vi "Instr Panel.vi"() -> ()   [LabVIEW 2009]
uses:
  Instruments/DAQ/DAQmx Analog.lvclass
  Instruments/Function Generator/Function Generator.lvclass
  Global/Flags.vi
  Main.vi
  Instruments/Utility Classes/Instrument/Instrument.lvclass
  File IO/File IO.lvclass
  Instruments/LCD/LCD Retarder.lvclass
  Instruments/Lockin/Lockin SR830.lvclass
  Instruments/Spectrometer/Spectrometer Triax 550.lvclass
  Instruments/Microwave/Microwave.lvclass
  Instruments/Pulse Gen/Pulse Generator.lvclass
  Instruments/Photon Counter/Photon Counter SR400.lvclass
  Instruments/Magnet/Power Supply/Power Supply.lvclass
panel:
  in  "Frequent\nReading":bool
  out "Find instruments (auto)":bool
  out "Status array":T1(array[cluster])
  in  "controlFMsweep":bool
  in  "Photon Counter":bool
  out "readtime":u32 caption="Read Time"
  in  "LDcontrol":bool
  in  "FGcontrol":bool
  in  "MWcontrol":bool
  in  "searchGPIB":bool
  in  "GPIB Comm.":bool
  in  "Find Instruments":bool
  in  "etchLD":bool
  in  "Open Driver":bool
  out "instrchecking":bool caption="Reading"
  in  "chop":bool
  in  "center-span":bool
  out "active":bool caption="Active"
  out "done":bool
  in  "exit":bool
  in  "Pulse Gen":bool
  in  "Magnet":bool
  in  "gotoLCD":bool
  in  "gotospect":bool
  # "On"
  # "Off"
  # "ms"
  # "Instruments Array"
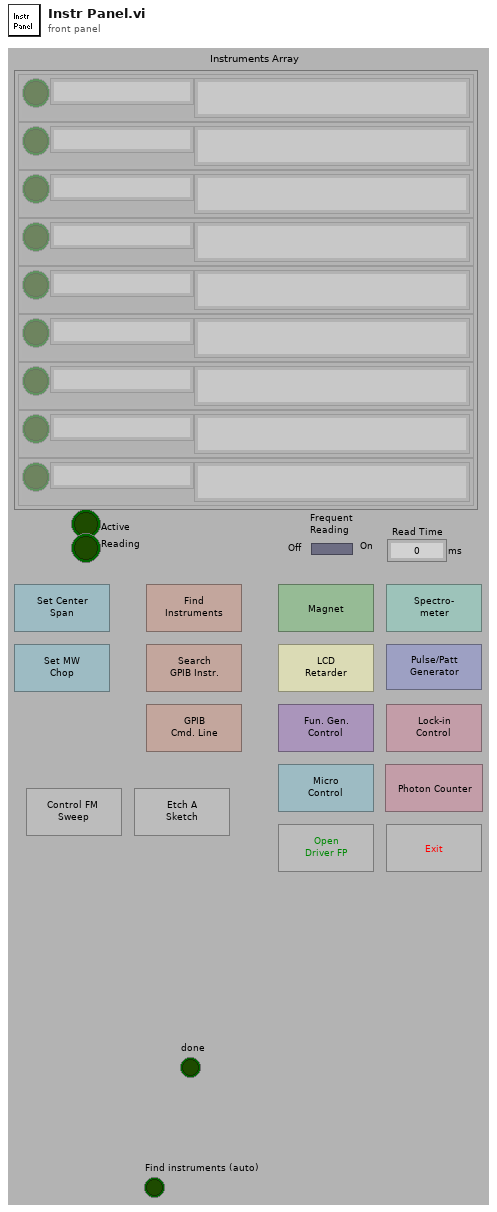
[diagram p1: front panel]
types:
  T1 = cluster{"On?":bool, "Name":string, "Status":string}[]
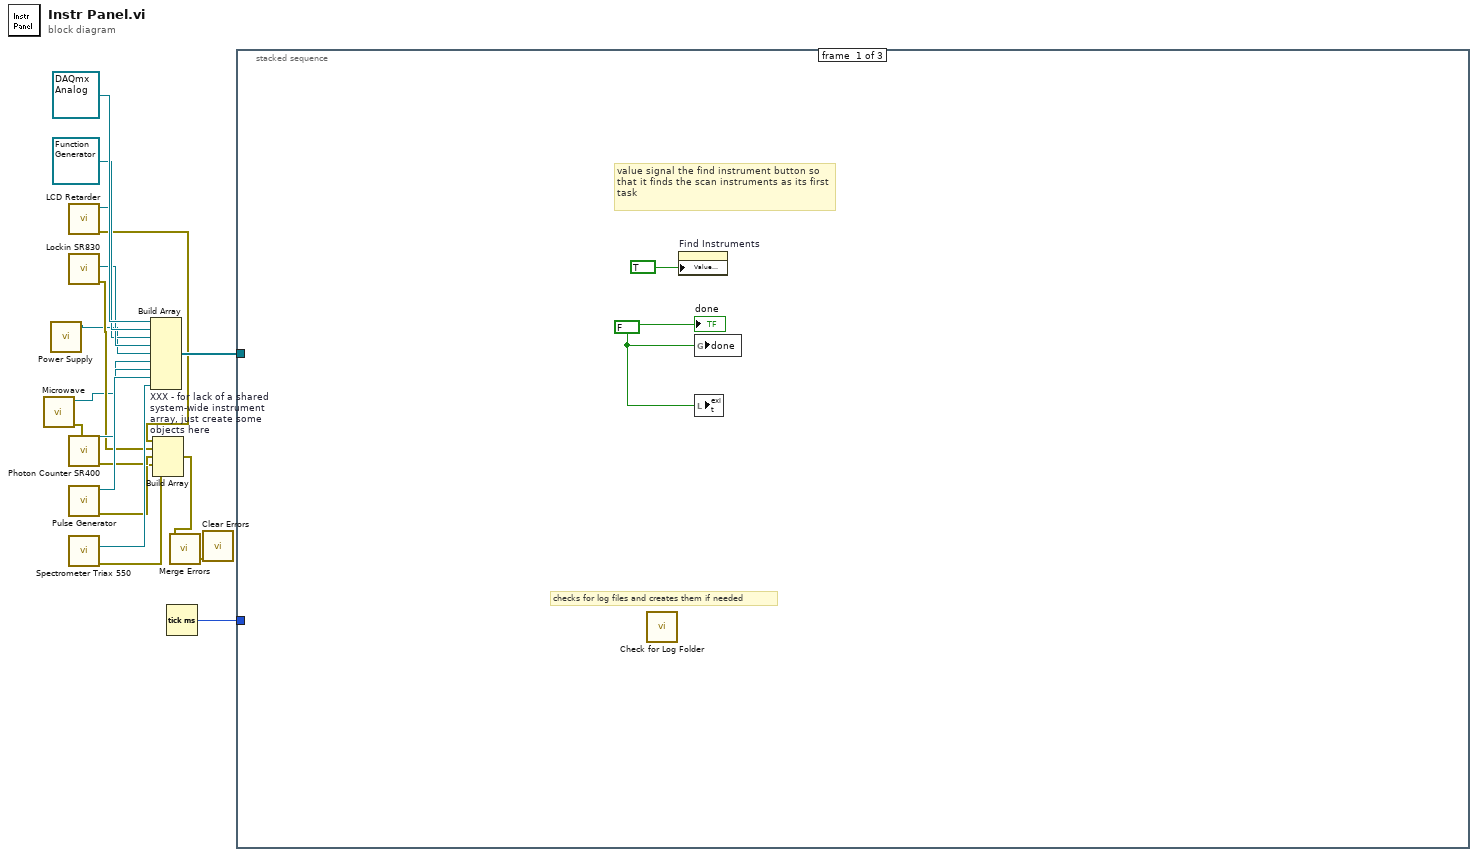
[diagram p0: block diagram]
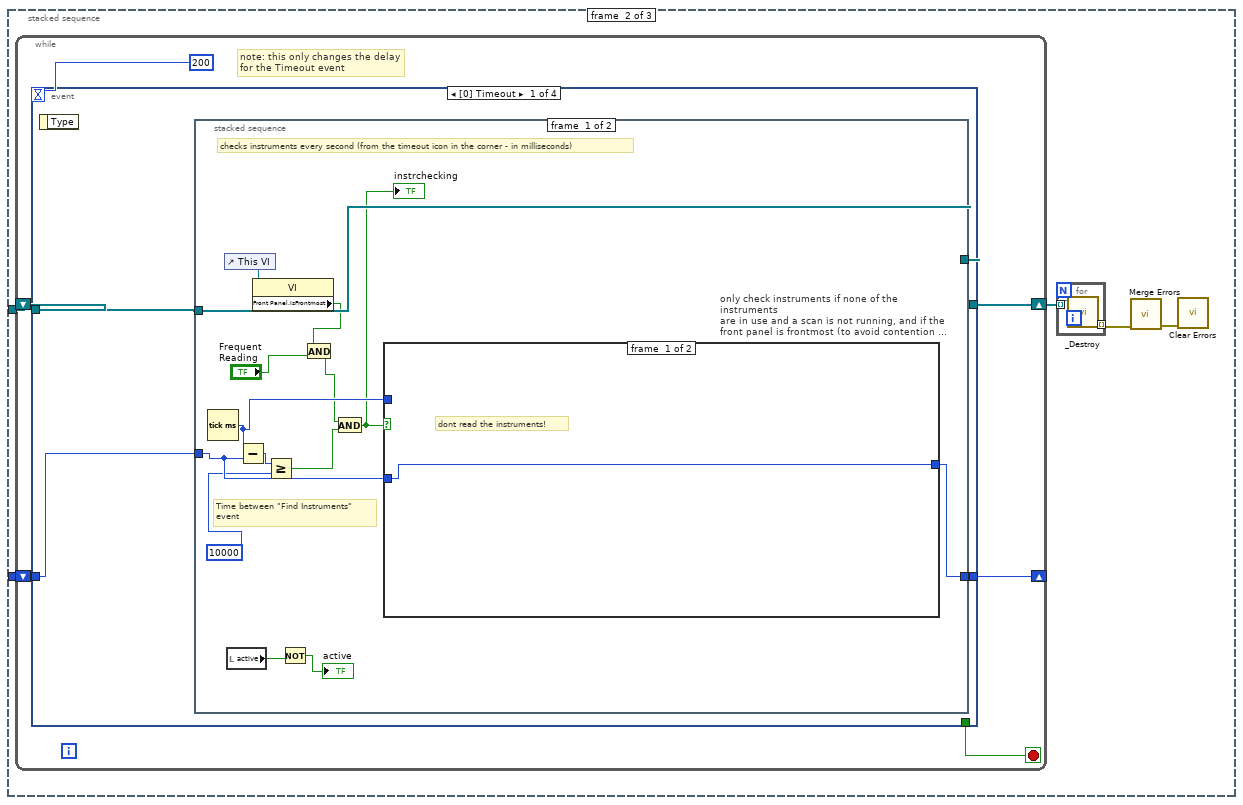
[diagram p2: hidden frame]
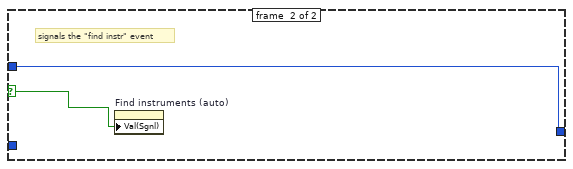
[diagram p3: hidden frame]
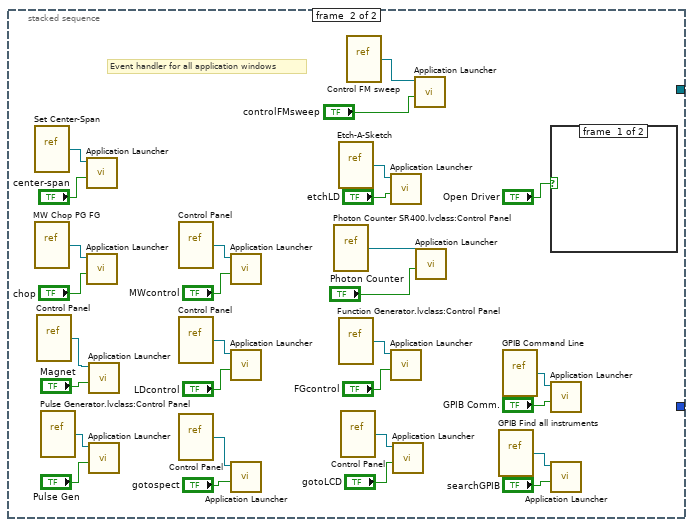
[diagram p4: hidden frame]
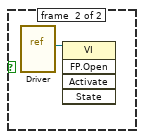
[diagram p5: hidden frame]
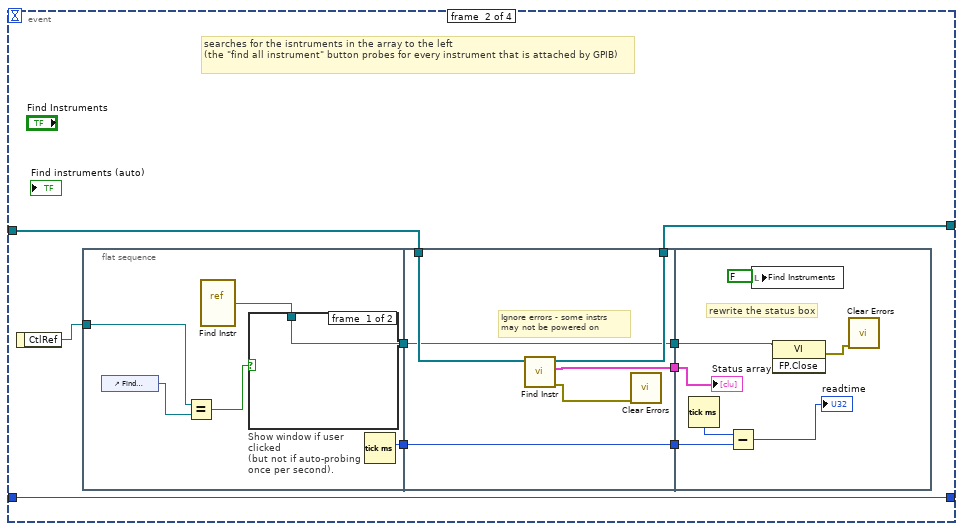
[diagram p6: hidden frame]
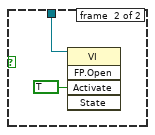
[diagram p7: hidden frame]
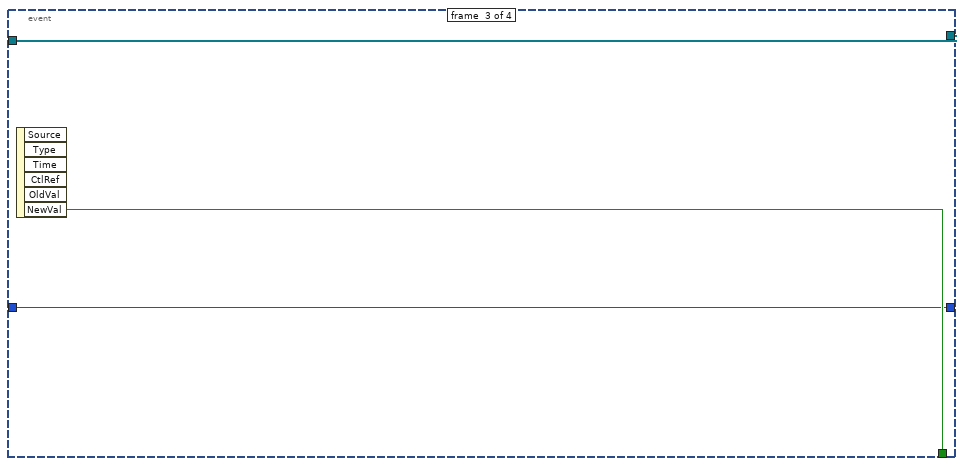
[diagram p8: hidden frame]
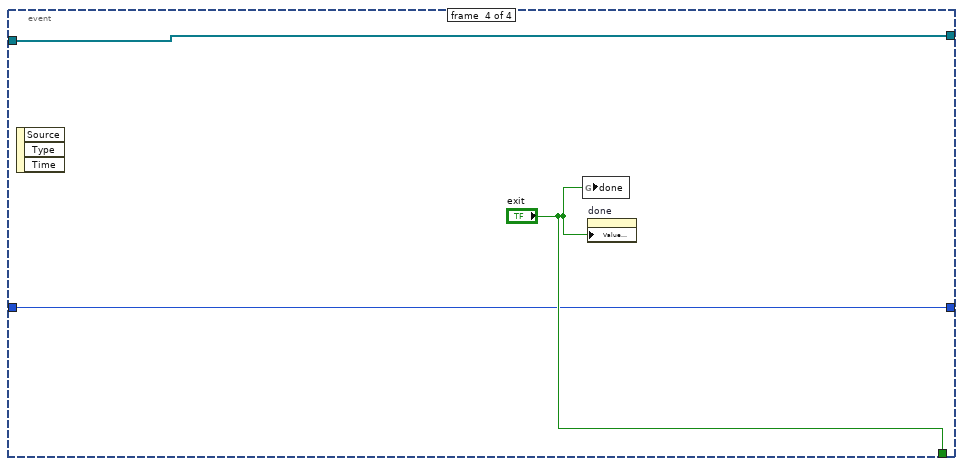
[diagram p9: hidden frame]
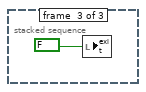
[diagram p10: hidden frame]
diagram:
  n1 = call "Microwave.vi"() -> ("error out"=w3:errorcluster, "Microwave out"=w2:refnum<class "Microwave.lvclass">)  [unwired: 10 in]
  n2 = call "Power Supply.vi"() -> ("Power Supply out"=w4:refnum<class "Power Supply.lvclass">)  [unwired: 10 in, 1 out]
  n3 = call "LCD Retarder.vi"() -> ("errorOUT"=w7:errorcluster, "LCD out"=w12:refnum<class "LCD Retarder.lvclass">)  [unwired: 1 in, 9 out]
  n4 = call "Lockin SR830.vi"() -> ("error out"=w8:errorcluster, "Lockin SR830 out"=w13:refnum<class "Lockin SR830.lvclass">)  [unwired: 1 in, 9 out]
  n5 = call "Photon Counter SR400.vi"("error in (no error)"=w3) -> ("error out"=w11:errorcluster, "Photon Counter SR400 out"=w14:refnum<class "Photon Counter SR400.lvclass">)  [unwired: 9 out]
  n6 = call "Pulse Generator.vi"() -> ("error out"=w10:errorcluster, "Pulse Generator out"=w16:refnum<class "Pulse Generator.lvclass">)  [unwired: 1 in, 9 out]
  n7 = call "Spectrometer Triax 550.vi"() -> ("error out"=w9:errorcluster, "Spectrometer Triax 550 out"=w15:refnum<class "Spectrometer Triax 550.lvclass">)  [unwired: 2 in, 8 out]
  n8 = Build Array "XXX - for lack of a shared\nsystem-wide instrument\narray, just create some\nobjects here"(refnum<class "DAQmx Analog.lvclass"> refnum ("DAQmx Analog.lvclass"), refnum<class "Function Generator.lvclass"> refnum ("Function Generator.lvclass"), w12, w13, w4, w2, w14, w16, w15) -> (w17:refnum<class "Instrument.lvclass">[])
  n9 = Build Array(w7, w8, w11, w10, w9) -> (w6:errorcluster[])
  n10 = Tick Count (ms)() -> (millisecond timer value=w1:u32)
  n11 = call <vilib>:"Merge Errors.vi"("error array in"=w6) -> ("error out"=w5:errorcluster)  [unwired: 3 in, 3 out]
  n12 = call <vilib>:"Clear Errors.vi"("error in (no error)"=w5) -> ()  [unwired: 7 out]
  n13 = stacked-sequence {
    tunnel: w17 -> [_ w26 _]
    tunnel: w1 -> [_ w22 _]
    frame #0 {
      w20 = FALSE
      # "value signal the find instrument button so that it finds the scan instruments as its first task"
      # "checks for log files and creates them if needed"
      n14 = call "Check for Log Folder.vi"() -> ()  [unwired: 1 out]
      n15 = property on="Find Instruments" class="Bool (strict)"("Value (Signaling)"=TRUE) -> ()  [unwired: 2 in, 2 out]
      n16 = global write "Flags.vi" "done"(w20) -> ()
      n17 = local write "exit"(w20) -> ()
      "done" <- w20
    }
    frame #1 {
      n18 = while {
        shift-right: [w31] -> w25
        shift-left: w26 -> [w32]
        shift-right: [w29] -> _
        shift-left: w22 -> [w30]
        stop <- w33 stop-if-true
        # "note: this only changes the delay \nfor the Timeout event"
        n19 = event shown="[0] Timeout" {
          selector: _ -> [_ _ _ _]
          dyn-events: _ -> [_ _ _ _]
          timeout: 200 -> [_ _ _ _]
          tunnel: [_ _ w117 "exit"] -> w33
          tunnel: w32 -> [w38 w94 w116 w119]
          tunnel: [w37 w93 w116 w119] -> w31
          tunnel: w30 -> [w36 w86 w115 w118]
          tunnel: [w35 w86 w115 w118] -> w29
          event #0 {
            n20 = event-data() -> ()  [unwired: 2 out]
            n21 = stacked-sequence {
              tunnel: w38 -> [w49 _]
              tunnel: [w49 _] -> w37
              tunnel: w36 -> [w44 _]
              tunnel: [w43 _] -> w35
              frame #0 {
                # "Time between \"Find Instruments\"\nevent"
                # "checks instruments every second (from the timeout icon in the corner - in milliseconds)"
                n22 = Tick Count (ms)() -> (millisecond timer value=w45:u32)
                n23 = control-ref of="This VI"() -> (w52:refnum<vi>)
                n24 = local read "active"() -> (w51:bool)
                n25 = Subtract(x=w45, y=w44) -> (x-y=w48:u32)
                n26 = property class="VI"(reference=w52) -> ("Front Panel.IsFrontmost"=w47:bool)  [unwired: 1 in, 2 out]
                n27 = Greater Or Equal?(x=w48, y=10000) -> (x >= y?=w46:bool)
                n28 = Not(x=w51) -> (.not. x?=→"active":bool)
                n29 = And(x=w47, y="Frequent\nReading") -> (x .and. y?=w41:bool)
                n30 = And(x=w41, y=w46) -> (x .and. y?=w42:bool)
                "instrchecking" <- w42
                n31 = case "only check instruments if none of the instruments \nare in use and a scan is not running, and if the \nfront panel is frontmost (to avoid contention on\n the GPIB bus when other VIs are running)" shown="False" w42 {
                  selector: w42 -> [_ w55]
                  tunnel: w45 -> [_ w54]
                  tunnel: w44 -> [w53 _]
                  tunnel: [w53 w54] -> w43
                  frame #0 {
                    # "dont read the instruments!"
                  }
                  frame #1 {
                    # "signals the \"find instr\" event"
                    n32 = property on="Find instruments (auto)" class="Bool (strict)"("Val(Sgnl)"=w55) -> ()  [unwired: 2 in, 2 out]
                  }
                }
              }
              frame #1 {
                # "Event handler for all application windows"
                n33 = vi-ref "Set Center-Span.vi"() -> (w84:refnum<vi>)
                n34 = vi-ref "MW Chop PG FG.vi"() -> (w82:refnum<vi>)
                n35 = vi-ref "Control Panel.vi"() -> (w61:refnum<vi>)
                n36 = vi-ref "Pulse Generator.lvclass:Control Panel.vi"() -> (w63:refnum<vi>)
                n37 = call "Application Launcher.vi"("Toggle?"="center-span", "VI reference"=w84) -> ()  [unwired: 2 in, 8 out]
                n38 = call "Application Launcher.vi"("Toggle?"="chop", "VI reference"=w82) -> ()  [unwired: 2 in, 8 out]
                n39 = call "Application Launcher.vi"("Toggle?"="Magnet", "VI reference"=w61) -> ()  [unwired: 2 in, 8 out]
                n40 = call "Application Launcher.vi"("Toggle?"="Pulse Gen", "VI reference"=w63) -> ()  [unwired: 2 in, 8 out]
                n41 = vi-ref "Control Panel.vi"() -> (w80:refnum<vi>)
                n42 = vi-ref "Control Panel.vi"() -> (w78:refnum<vi>)
                n43 = vi-ref "Control Panel.vi"() -> (w70:refnum<vi>)
                n44 = call "Application Launcher.vi"("Toggle?"="MWcontrol", "VI reference"=w80) -> ()  [unwired: 2 in, 8 out]
                n45 = call "Application Launcher.vi"("Toggle?"="LDcontrol", "VI reference"=w78) -> ()  [unwired: 2 in, 8 out]
                n46 = call "Application Launcher.vi"("Toggle?"="gotospect", "VI reference"=w70) -> ()  [unwired: 2 in, 8 out]
                n47 = vi-ref "Photon Counter SR400.lvclass:Control Panel.vi"() -> (w59:refnum<vi>)
                n48 = vi-ref "Etch-A-Sketch.vi"() -> (w68:refnum<vi>)
                n49 = vi-ref "Function Generator.lvclass:Control Panel.vi"() -> (w76:refnum<vi>)
                n50 = vi-ref "Control Panel.vi"() -> (w72:refnum<vi>)
                n51 = vi-ref "Control FM sweep.vi"() -> (w56:refnum<vi>)
                n52 = call "Application Launcher.vi"("Toggle?"="etchLD", "VI reference"=w68) -> ()  [unwired: 1 in, 9 out]
                n53 = call "Application Launcher.vi"("Toggle?"="FGcontrol", "VI reference"=w76) -> ()  [unwired: 2 in, 8 out]
                n54 = call "Application Launcher.vi"("Toggle?"="gotoLCD", "VI reference"=w72) -> ()  [unwired: 2 in, 8 out]
                n55 = call "Application Launcher.vi"("Toggle?"="controlFMsweep", "VI reference"=w56) -> ()  [unwired: 1 in, 9 out]
                n56 = call "Application Launcher.vi"("Toggle?"="Photon Counter", "VI reference"=w59) -> ()  [unwired: 2 in, 8 out]
                n57 = vi-ref "GPIB Find all instruments.vi"() -> (w74:refnum<vi>)
                n58 = vi-ref "GPIB Command Line.vi"() -> (w65:refnum<vi>)
                n59 = case shown="True" "Open Driver" {
                  frame #0 {
                  }
                  frame #1 {
                    n60 = vi-ref "Driver.vi"() -> (w85:refnum<vi>)
                    n61 = invoke class="VI" method="FP.Open"(reference=w85) -> ()  [unwired: 4 in, 5 out]
                  }
                }
                n62 = call "Application Launcher.vi"("Toggle?"="GPIB Comm.", "VI reference"=w65) -> ()  [unwired: 1 in, 9 out]
                n63 = call "Application Launcher.vi"("Toggle?"="searchGPIB", "VI reference"=w74) -> ()  [unwired: 1 in, 9 out]
              }
            }
          }
          event #1 {
            # "searches for the isntruments in the array to the left \n(the \"find all instrument\" button probes for every instrument that is attached by GPIB)"
            n64 = event-data() -> ("CtlRef"=w92:refnum<vi>)  [unwired: 1 out]
            n65 = flat-sequence {
              tunnel: [w99] -> w91
              tunnel: w92 -> [w97]
              tunnel: [w98] -> w90
              tunnel: [w107] -> w89
              tunnel: w91 -> [w107]
              tunnel: w94 -> [w106]
              tunnel: [w105] -> w93
              tunnel: [w103] -> w88
              tunnel: [w102] -> w87
              tunnel: w90 -> [w102]
              tunnel: w89 -> [w113]
              tunnel: w88 -> [w111]
              tunnel: w87 -> [w110]
              frame #0 {
                n66 = control-ref of="Find Instruments"() -> (w95:refnum<vi>)
                n67 = Equal?(x=w97, y=w95) -> (x = y?=w96:bool)
                n68 = vi-ref "Find Instr.vi"() -> (w98:refnum<vi>)
                n69 = case "Show window if user clicked\n(but not if auto-probing\nonce per second)." shown="True" w96 {
                  tunnel: w98 -> [_ w101]
                  frame #0 {
                  }
                  frame #1 {
                    n70 = invoke class="VI" method="FP.Open"(reference=w101, "Activate"=TRUE ("Activate?")) -> ()  [unwired: 3 in, 5 out]
                  }
                }
                n71 = Tick Count (ms)() -> (millisecond timer value=w99:u32)
              }
              frame #1 {
                # "Ignore errors - some instrs\nmay not be powered on"
                n72 = call "Find Instr.vi"("Instrument array"=w106) -> ("error out"=w104:errorcluster, "Status array"=w103:T1, "Instrument array out"=w105:refnum<class "Instrument.lvclass">[])  [unwired: 1 in, 7 out]
                n73 = call <vilib>:"Clear Errors.vi"("error in (no error)"=w104) -> ()  [unwired: 7 out]
              }
              frame #2 {
                # "rewrite the status box"
                n74 = Tick Count (ms)() -> (millisecond timer value=w114:u32)
                n75 = Subtract(x=w114, y=w113) -> (x-y=→"readtime":u32)
                n76 = local write "Find Instruments"(FALSE) -> ()
                n77 = invoke class="VI" method="FP.Close"(reference=w110) -> (error out=w109:errorcluster)  [unwired: 2 in, 2 out]
                n78 = call <vilib>:"Clear Errors.vi"("error in (no error)"=w109) -> ()  [unwired: 7 out]
                "Status array" <- w111
              }
            }
          }
          event #2 {
            n79 = event-data() -> ("NewVal"=w117:bool)  [unwired: 6 out]
          }
          event #3 {
            n80 = event-data() -> ()  [unwired: 4 out]
            n81 = global write "Flags.vi" "done"("exit") -> ()
            n82 = property on="done" class="Boolean (strict)"("Value (Signaling)"="exit") -> ()  [unwired: 2 in, 2 out]
          }
        }
      }
      n83 = for {
        tunnel: w25 -> [w28] mode=indexing
        tunnel: [w27] -> w24 mode=indexing
        n84 = call-dynamic "_Destroy.vi"("Instrument in"=w28) -> ("error out"=w27:errorcluster)  [unwired: 1 in, 9 out]
      }
      n85 = call <vilib>:"Merge Errors.vi"("error array in"=w24) -> ("error out"=w23:errorcluster)  [unwired: 3 in, 3 out]
      n86 = call <vilib>:"Clear Errors.vi"("error in (no error)"=w23) -> ()  [unwired: 7 out]
    }
    frame #2 {
      n87 = local write "exit"(FALSE) -> ()
    }
  }
